vi "ContinueScan.vi"(10 "input cluster":T1={"Scanning Segments Left"=0, "Scanning"=FALSE, "Path"=path "", "FileName"="", "Scan Segments"=0, "Step Time (us)"=100, "Polarity"=enum."Positive", "Direction"=enum."Forward", "Steps"=1} {"Steps" min=1 max=10000 step=1 scale=1.0..10000.0; "Step Time (us)" min=100 step=10 scale=100.0..10000.0; "Scan Segments" max=100 step=1 scale=0.0..100.0}, 11 "Message Enqueuer in":refnum<class "Message Enqueuer.lvclass">) -> (2 "output cluster":T1={"Scanning Segments Left"=0, "Scanning"=FALSE, "Path"=path "", "FileName"="", "Scan Segments"=0, "Step Time (us)"=100, "Polarity"=enum."Positive", "Direction"=enum."Forward", "Steps"=1} {"Steps" min=1 max=10000 step=1 scale=1.0..10000.0; "Step Time (us)" min=100 step=10 scale=100.0..10000.0; "Scan Segments" max=100 step=1 scale=0.0..100.0})   [LabVIEW 2023, in "InterferometryUI.lvlib" / "InterferometryUI.lvclass"]
uses:
  InterferometryUI.lvclass
  ArduinoTranslationStageUI/ArduinoTranslationStageActor/ArduinoTranslationStage Messages/MoveBySteps Msg/MoveBySteps Msg.lvclass
  <vilib>/ActorFramework/Message Enqueuer/Message Enqueuer.lvclass
  InterferometryUIPublicData.ctl
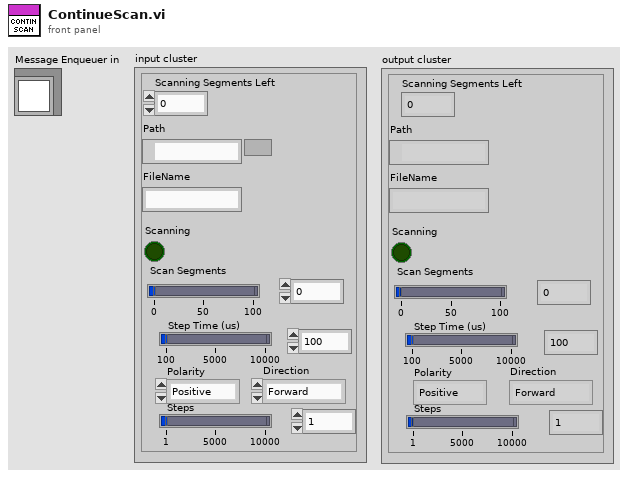
[diagram p1: front panel]
types:
  T1 = typedef "InterferometryUIPublicData.ctl" = cluster{"Scanning Segments Left":u16, "Scanning":bool, "Path":path, "FileName":string, "Scan Segments":u32, "Step Time (us)":u32, "Polarity":enum16{"Positive", "Negative"}, "Direction":enum16{"Forward", "Backwards"}, "Steps":u32}
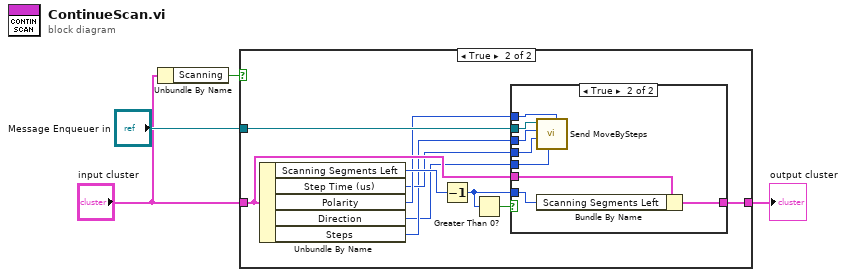
[diagram p0: block diagram]
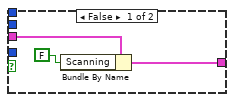
[diagram p3: hidden frame]
diagram:
  n1 = Unbundle By Name("input cluster") -> ("Scanning"=w3:bool)
  n2 = case shown="True" w3 {
    tunnel: [w5 w15] -> w1
    tunnel: "Message Enqueuer in" -> [_ w12]
    tunnel: "input cluster" -> [w5 w10]
    frame False {
    }
    frame True {
      n3 = Unbundle By Name(w10) -> ("Scanning Segments Left"=w11:u16, "Step Time (us)"=w8:u32, "Polarity"=w9:enum16{"Positive", "Negative"}, "Direction"=w6:enum16{"Forward", "Backwards"}, "Steps"=w7:u32)
      n4 = Decrement(x=w11) -> (x-1=w14:u16)
      n5 = Greater Than 0?(x=w14) -> (x > 0?=w13:bool)
      n6 = case shown="True" w13 {
        tunnel: [w17 w20] -> w15
        tunnel: w14 -> [_ w26]
        tunnel: w12 -> [_ w25]
        tunnel: w10 -> [w16 w19]
        tunnel: w9 -> [_ w24]
        tunnel: w8 -> [_ w23]
        tunnel: w7 -> [_ w22]
        tunnel: w6 -> [_ w21]
        frame False {
          n7 = Bundle By Name(cluster=w16, "Scanning"=FALSE) -> (w17:T1)
        }
        frame True {
          n8 = call "Send MoveBySteps.vi"("Polarity"=w24, "Direction"=w21, "Speed"=w23, "Steps"=w22, "Message Enqueuer"=w25) -> ()  [unwired: 5 in, 2 out]
          n9 = Bundle By Name(cluster=w19, "Scanning Segments Left"=w26) -> (w20:T1)
        }
      }
    }
  }
  "output cluster" <- w1
